vi "GestioneFernoSubVI2.vi"(0 "Cluster in":refnum<vi>, 1 "reference 3":refnum<vi>, 2 "reference 4":refnum<vi>, 3 "reference 5":refnum<vi>, 4 "Bool Refnum":refnum<vi>, 5 "reference 6":refnum<vi>, 6 "Clust Refnum":refnum<vi>, 8 "reference in":refnum<vi>, 9 "Clust Refnum 2":refnum<vi>, 10 "Array stato freni":T1[](array[typedef]) {"Rif AO coppia freno[Nm]" format="%#_13g"}, 11 "reference 7":refnum<vi>, 12 "Numeric in":dbl, 13 "reference 8":refnum<vi>, 14 "Numeric in":dbl, 15 "reference 9":refnum<vi>, 16 "Freno selezionato":i32) -> (18 "DI senso rotaz freno":bool, 20 "Boolean":bool, 21 "Gestione freno":T2, 22 "Running":bool)   [LabVIEW 2019]
uses:
  TypeDef/Comandi freno.ctl
  TypeDef/Stato_inverter.ctl
  TypeDef/Stato inverter selezionato.ctl
  Stato alimentatore 1.vi
  Global CTRL VELOCITA.vi
  Stato comandi freno.vi
  Global FINE AVVIO.vi
panel:
  # "CHANGING CONTROL\nTYPE...."
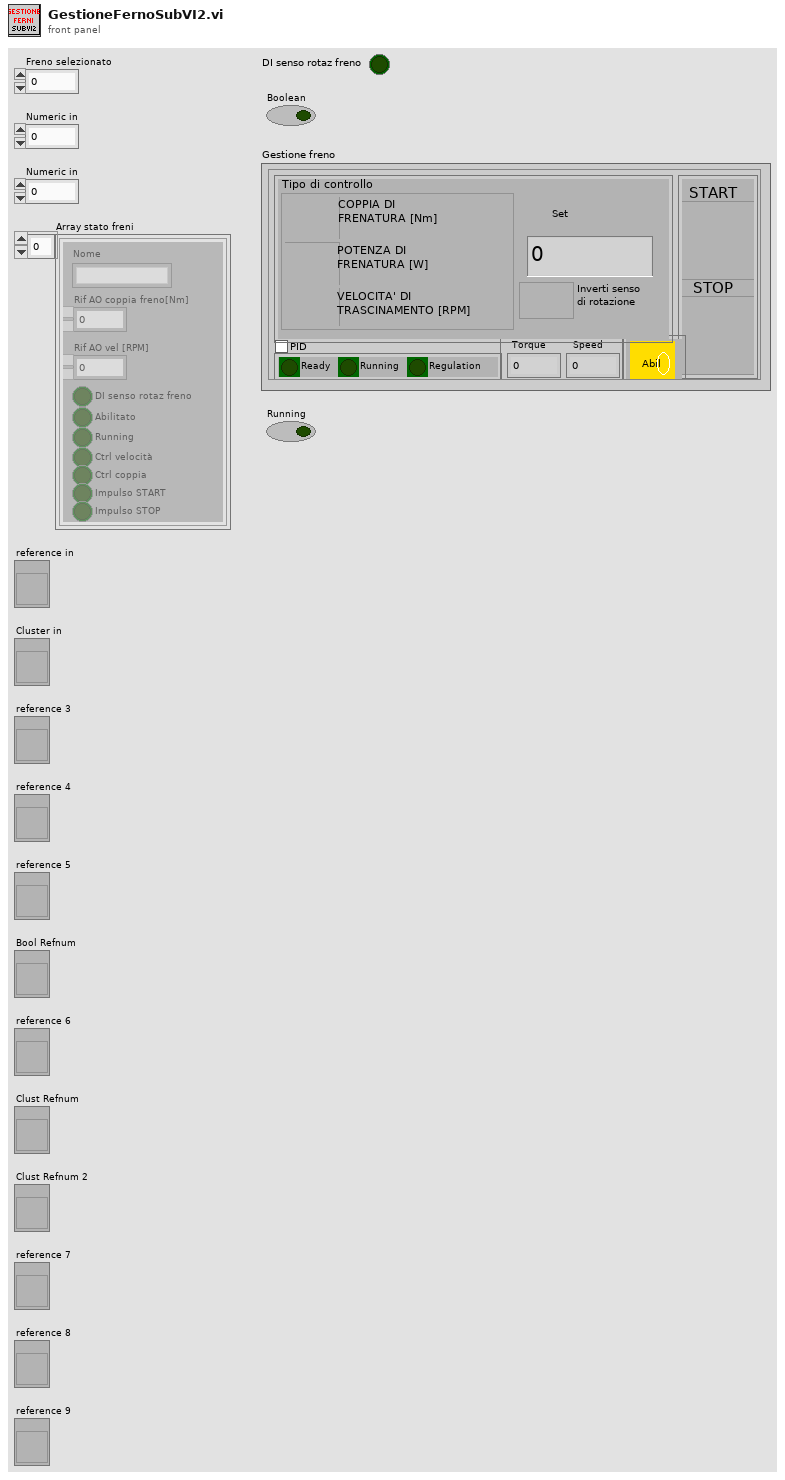
[diagram p1: front panel]
types:
  T1 = typedef "Stato_inverter.ctl" = cluster{"DI senso rotaz freno":bool, "Rif AO vel [RPM]":dbl, "Rif AO coppia freno[Nm]":dbl, "Abilitato":bool, "Running":bool, "Ctrl velocità":bool, "Nome":string, "Ctrl coppia":bool, "Impulso START":bool, "Impulso STOP":bool}
  T2 = typedef "Comandi freno.ctl" = cluster{"Control":cluster{"Control Type":enum32{"Torque [Nm]", "Power [W]", "Speed [RPM]"}, "Set":dbl, "Inverti senso di rotazione":bool}, "Start\\stop":cluster{"Start":bool, "STOP":bool}, "Status":cluster{"Ready":bool, "Running":bool, "Regulation":bool}, "PID":bool, "Abilita":cluster{"Abilita":bool}, "Status ref":cluster{"Torque":dbl, "Speed":dbl}}
  T3 = typedef "Stato inverter selezionato.ctl" = cluster{"Stato comandi freno":T2, "Stato":cluster{"rif C%":dbl, "rif vel%":dbl, "Controllo effettivo":enum32{"Torque [Nm]", "Power [W]", "Speed [RPM]"}, "Controllo desiderato":enum32{"Torque [Nm]", "Power [W]", "Speed [RPM]"}, "Fine rampa C":bool, "Fine rampa RPM":bool, "Senso rotaz":bool, "Start":bool, "C stabile":bool, "P stabile":bool, "RPM stabile":bool}}
  T4 = enum32{"Torque [Nm]", "Power [W]", "Speed [RPM]"}
  T5 = typedef "Comandi_Alimentatore.ctl" = cluster{"RIF 1":dbl, "RIF 2":dbl, "Status":cluster{"Ready":bool, "Running":bool, "Regulation":bool}, "Start\\stop":cluster{"Start":bool, "Stop":bool}, "PID RIF1":bool, "PID RIF2":bool, "Status ref":cluster{"RIF 1":dbl, "RIF 2":dbl}, "Abilita":cluster{"Abilita":bool}}
  T6 = cluster{"RIF 1":dbl, "RIF 2":dbl, "Abilitato":bool, "In marcia":bool, "Fine rampa RIF1":bool, "Fine rampa RIF2":bool, "Vstabile":bool, "F stabile":bool, "PID RIF1":bool, "PID RIF2":bool, "Alimentatore 1":T5}
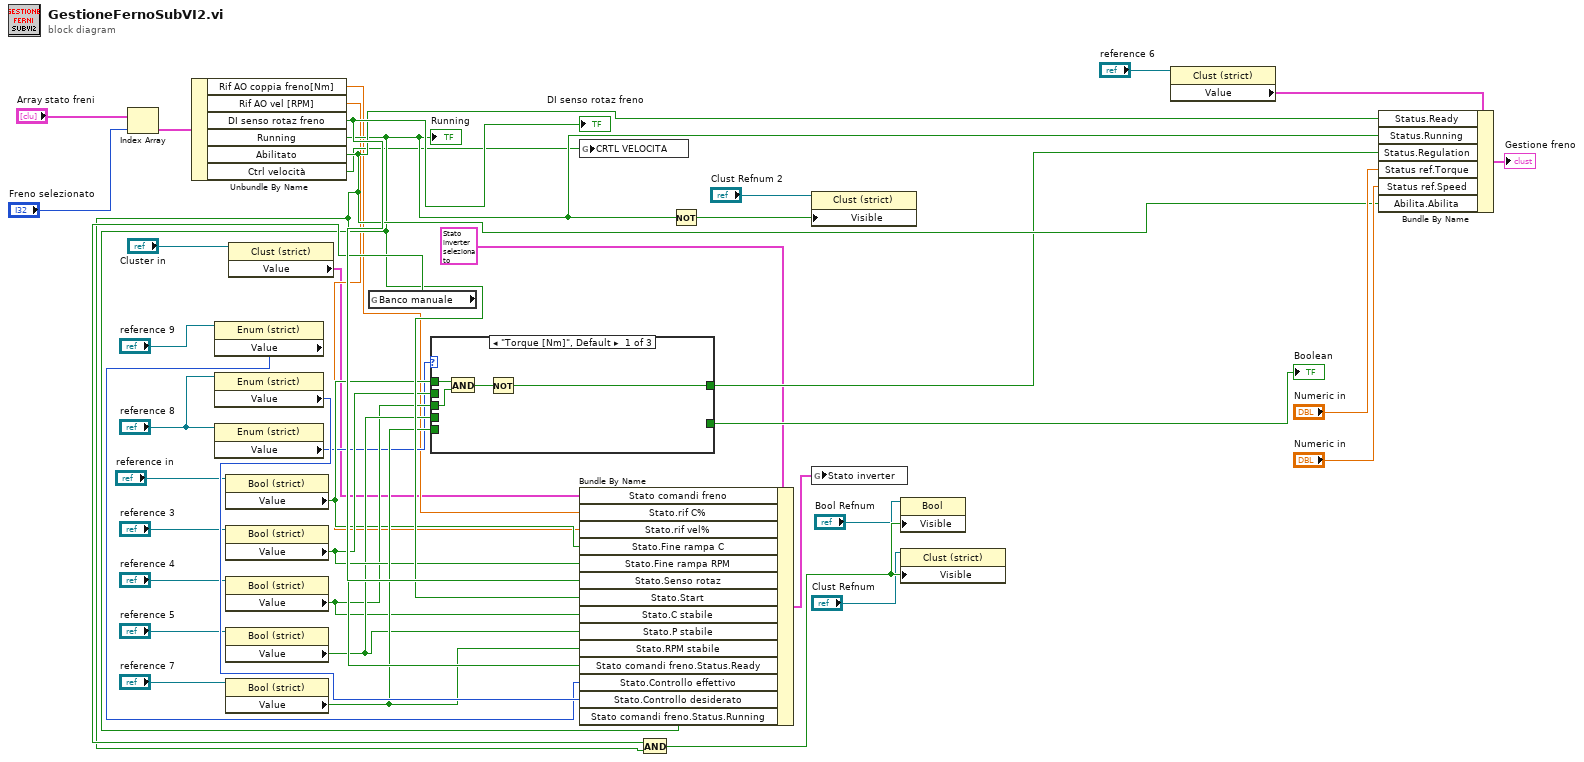
[diagram p0: block diagram]
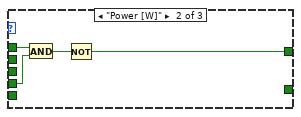
[diagram p2: hidden frame]
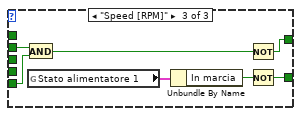
[diagram p3: hidden frame]
diagram:
  n1 = Index Array(array="Array stato freni", index="Freno selezionato") -> (element=w13:T1)
  n2 = Unbundle By Name(w13) -> ("Rif AO coppia freno[Nm]"=w21:dbl, "Rif AO vel [RPM]"=w22:dbl, "DI senso rotaz freno"=w41:bool, "Running"=w34:bool, "Abilitato"=w36:bool, "Ctrl velocità"=w24:bool)
  "DI senso rotaz freno" <- w41
  "Running" <- w34
  n3 = property class="Enum (strict)"(reference="reference 9") -> ("Value"=w32:T4)  [unwired: 1 in, 2 out]
  n4 = property class="Enum (strict)"(reference="reference 8") -> ("Value"=w33:T4)  [unwired: 1 in, 2 out]
  n5 = property class="Enum (strict)"(reference="reference 8") -> ("Value"=w25:T4)  [unwired: 1 in, 2 out]
  n6 = property class="Bool (strict)"(reference="reference in") -> ("Value"=w26:bool)  [unwired: 1 in, 2 out]
  n7 = property class="Bool (strict)"(reference="reference 3") -> ("Value"=w30:bool)  [unwired: 1 in, 2 out]
  n8 = property class="Bool (strict)"(reference="reference 4") -> ("Value"=w27:bool)  [unwired: 1 in, 2 out]
  n9 = property class="Bool (strict)"(reference="reference 5") -> ("Value"=w29:bool)  [unwired: 1 in, 2 out]
  n10 = property class="Bool (strict)"(reference="reference 7") -> ("Value"=w31:bool)  [unwired: 1 in, 2 out]
  n11 = property class="Clust (strict)"(reference="Cluster in") -> ("Value"=w15:T2)  [unwired: 1 in, 2 out]
  n12 = global read "Global FINE AVVIO.vi" "Banco manuale"() -> (w38:bool)
  n13 = case shown="\"Torque [Nm]\", Default" w25 {
    tunnel: w26 -> [w44 w49 _]
    tunnel: w27 -> [w45 _ _]
    tunnel: [w42 w46 w53] -> w28
    tunnel: w29 -> [_ w48 _]
    tunnel: w30 -> [_ _ w56]
    tunnel: w31 -> [_ _ w55]
    tunnel: [_ _ w50] -> w35
    frame "Torque [Nm]", Default {
      n14 = And(x=w44, y=w45) -> (x .and. y?=w43:bool)
      n15 = Not(x=w43) -> (.not. x?=w42:bool)
    }
    frame "Power [W]" {
      n16 = And(x=w49, y=w48) -> (x .and. y?=w47:bool)
      n17 = Not(x=w47) -> (.not. x?=w46:bool)
    }
    frame "Speed [RPM]" {
      n18 = And(x=w56, y=w55) -> (x .and. y?=w54:bool)
      n19 = global read "Stato alimentatore 1.vi" "Stato alimentatore 1"() -> (w52:T6)
      n20 = Unbundle By Name(w52) -> ("In marcia"=w51:bool)
      n21 = Not(x=w54) -> (.not. x?=w53:bool)
      n22 = Not(x=w51) -> (.not. x?=w50:bool)
    }
  }
  "Boolean" <- w35
  n23 = global write "Global CTRL VELOCITA.vi" "CRTL VELOCITA"(w24) -> ()
  n24 = Bundle By Name(cluster=T3 {"Stato comandi freno"={"Control"={"Control Type"=enum."Torque [Nm]", "Set"=0.0, "Inverti senso di rotazione"=FALSE}, "Start\\stop"={"Start"=FALSE, "STOP"=FALSE}, "Status"={"Ready"=FALSE, "Running"=FALSE, "Regulation"=FALSE}, "PID"=FALSE, "Abilita"={"Abilita"=FALSE}, "Status ref"={"Torque"=0.0, "Speed"=0.0}}, "Stato"={"rif C%"=0.0, "rif vel%"=0.0, "Controllo effettivo"=enum."Torque [Nm]", "Controllo desiderato"=enum."Torque [Nm]", "Fine rampa C"=FALSE, "Fine rampa RPM"=FALSE, "Senso rotaz"=FALSE, "Start"=FALSE, "C stabile"=FALSE, "P stabile"=FALSE, "RPM stabile"=FALSE}} ("Stato inverter"), "Stato comandi freno"=w15, "Stato.rif C%"=w21, "Stato.rif vel%"=w22, "Stato.Fine rampa C"=w26, "Stato.Fine rampa RPM"=w30, "Stato.Senso rotaz"=w41, "Stato.Start"=w34, "Stato.C stabile"=w27, "Stato.P stabile"=w29, "Stato.RPM stabile"=w31, "Stato comandi freno.Status.Ready"=w36, "Stato.Controllo effettivo"=w32, "Stato.Controllo desiderato"=w33, "Stato comandi freno.Status.Running"=w34) -> (w16:T3)
  n25 = And(x=w38, y=w36) -> (x .and. y?=w40:bool)
  n26 = Not(x=w34) -> (.not. x?=w23:bool)
  n27 = property on="Property Node" class="Clust (strict)"(reference="Clust Refnum 2", "Visible"=w23) -> ()  [unwired: 1 in, 2 out]
  n28 = global write "Stato comandi freno.vi" "Stato inverter"(w16) -> ()
  n29 = property on="Property Node" class="Bool"(reference="Bool Refnum", "Visible"=w40) -> ()  [unwired: 1 in, 2 out]
  n30 = property on="Property Node" class="Clust (strict)"(reference="Clust Refnum", "Visible"=w40) -> ()  [unwired: 1 in, 2 out]
  n31 = property class="Clust (strict)"(reference="reference 6") -> ("Value"=w19:T2)  [unwired: 1 in, 2 out]
  n32 = Bundle By Name(cluster=w19, "Status.Ready"=w36, "Status.Running"=w34, "Status.Regulation"=w28, "Status ref.Torque"="Numeric in", "Status ref.Speed"="Numeric in", "Abilita.Abilita"=w36) -> (→"Gestione freno":T2)
